vi "Windows.Exit.vi"(7 "Exit Action":T1=enum."Shut Down PC") -> (0 "error out":errorcluster)   [LabVIEW 2016]
doc: "This VI allows you to exit windows in various ways.\nexit windows function\n0: Log off\n1: Shut Down\n2: Exit Windows and reboot the computer"
uses:
  Windows.ExitAction.ctl
  user32.dll
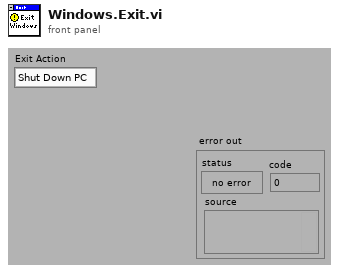
[diagram p1: front panel]
types:
  T1 = typedef "Windows.ExitAction.ctl" = enum16{"Log off from PC", "Shut Down PC", "Reboot PC", "Close Program"}
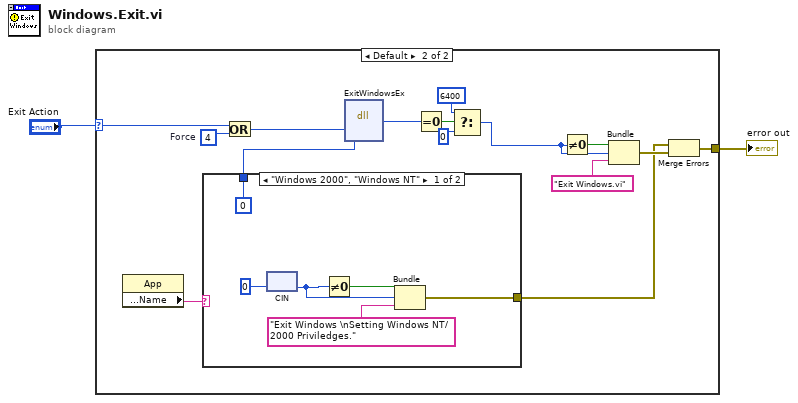
[diagram p0: block diagram]
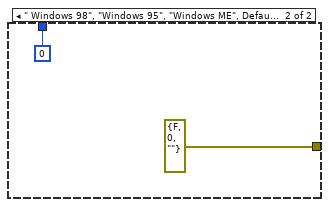
[diagram p3: hidden frame]
diagram:
  n1 = case shown="Default" "Exit Action" {
    selector: "Exit Action" -> [_ w3]
    tunnel: [_ w14] -> w2
    frame "Close Program" {
    }
    frame Default {
      w7 = u32 4  # Force
      n2 = property class="App"() -> ("Operating System:Name"=w5:string)  [unwired: 2 in, 2 out]
      n3 = case shown="\"Windows 2000\", \"Windows NT\"" w5 {
        tunnel: [u32 0 u32 0] -> w4
        tunnel: [w18 errorcluster {FALSE, 0, ""} ("Output Cluster")] -> w12
        frame "Windows 2000", "Windows NT" {
          n4 = cin(0) -> (w20:i32)
          n5 = Not Equal To 0?(x=w20) -> (x != 0?=w21:bool)
          n6 = Bundle(w21, w20, "Exit Windows \nSetting Windows NT/2000 Priviledges.") -> (w18:errorcluster)  [unwired: 1 out]
        }
        frame " Windows 98", "Windows 95", "Windows ME", Default {
        }
      }
      n7 = Or(x=w3, y=w7) -> (x .or. y?=w6:u32)
      n8 = dll-call lib="User32.dll" fn="ExitWindowsEx" label="ExitWindows"("returnCode"=w6, "reserved (set to zero)"=w4) -> (w8:i32)  [unwired: 5 in, 2 out]
      n9 = Equal To 0?(x=w8) -> (x = 0?=w9:bool)
      n10 = Select(t=6400, s=w9, f=0) -> (s? t:f=w16:i32)
      n11 = Not Equal To 0?(x=w16) -> (x != 0?=w17:bool)
      n12 = Bundle(w17, w16, "Exit Windows.vi") -> (w13:errorcluster)  [unwired: 1 out]
      n13 = Merge Errors(w12, w13) -> (w14:errorcluster)
    }
  }
  "error out" <- w2
